vi "Test Channel Configuration.vi"() -> ()   [LabVIEW 2013, in "fixed module parent tests.lvlib"]
uses:
  fixed module parent tests.lvlib
  module/configuration/fixed channel configuration.lvclass
  <vilib>/NI/Tag Bus/tag/tag descriptor.lvclass/tag descriptor.ctl
  <vilib>/NI/Tag Bus/tag/tag descriptor.lvclass
panel:
  out "Errors or Warnings in Creating Channels":errorcluster
  out "Channels that were configured correctly":string[](array[string])
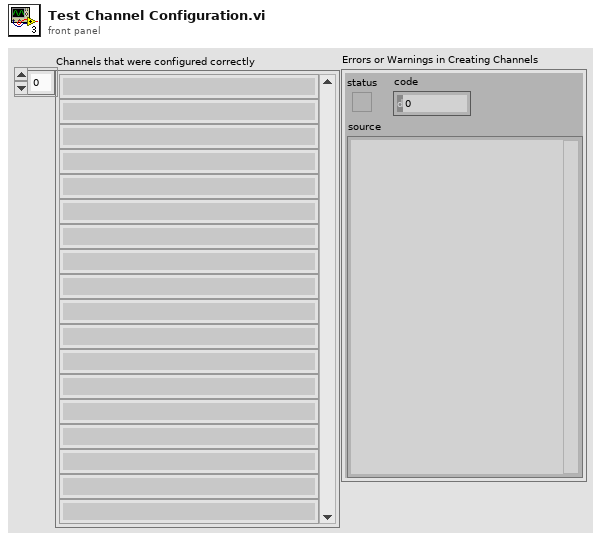
[diagram p1: front panel]
types:
  T1 = typedef "tag bus.lvlib/tag descriptor.lvclass/Data Type.ctl" = enum16{"Double", "Single", "I64", "I32", "I16", "I8", "U64", "U32", "U16", "U8", "Boolean", "String", "Array of Double", "Array of Single", "Array of I64", "Array of I32", "Array of I16", "Array of I8", "Array of U64", "Array of U32", "Array of U16", "Array of U8", "Array of Boolean", "Array of String"}
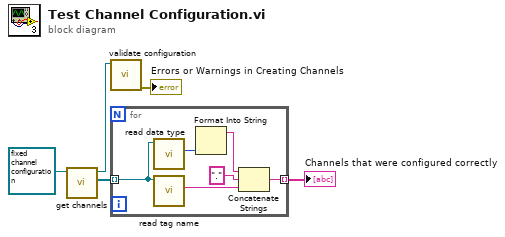
[diagram p0: block diagram]
diagram:
  n1 = call-dynamic "get channels.vi"("fixed module parent implementation configuration in"=refnum<class "fixed channel configuration.lvclass"> refnum ("user module configuration")) -> ("channels"=w3:refnum<class "TBM channel.lvclass">[], "fixed module parent implementation configuration out"=w4:refnum<class "fixed channel configuration.lvclass">)  [unwired: 9 in]
  n2 = call-dynamic "validate configuration.vi"("fixed module parent implementation configuration in"=w4) -> ("error out"=→"Errors or Warnings in Creating Channels":errorcluster)  [unwired: 9 in, 1 out]
  n3 = for {
    tunnel: w3 -> [w11] mode=indexing
    tunnel: [w8] -> w2 mode=indexing
    n4 = call <vilib>:"read data type.vi"("system tag in"=w11) -> ("data type"=w6:T1)  [unwired: 8 in, 2 out]
    n5 = call <vilib>:"read tag name.vi"("system tag in"=w11) -> ("name"=w7:string)  [unwired: 8 in, 2 out]
    n6 = Format Into String(w6) -> (resulting string=w9:string)  [unwired: 3 in, 1 out]
    n7 = Concatenate Strings(w9, "." ("resulting string"), w7) -> (w8:string)
  }
  "Channels that were configured correctly" <- w2
